vi "run_python_script_demoinfocom.vi"() -> ()   [LabVIEW 2021]
panel:
  in  "b":dbl
  out "c":i32
  in  "a":dbl
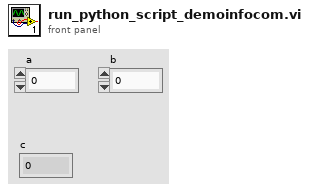
[diagram p1: front panel]
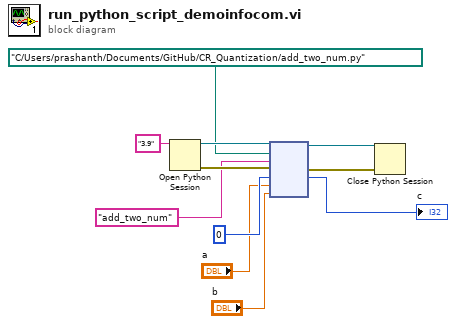
[diagram p0: block diagram]
diagram:
  n1 = Open Python Session(python version="3.9" ("Python version")) -> (session out=w11:refnum<k35>, error out=w9:errorcluster)  [unwired: 2 in]
  n2 = node ("Python Node")(w11, path "C:/Users/prashanth/Documents/GitHub/CR_Quantization/add_two_num.py" ("module path"), "add_two_num" ("function name"), w9, 0, "a", "b") -> (w10:refnum<k35>, w8:errorcluster, →"c":i32)  [unwired: 2 in, 2 out]
  n3 = Close Python Session(session in=w10, error in=w8) -> ()  [unwired: 1 out]
